vi "Generate ramp lists.vi"(9 "SMU2 settings":T1, 10 "SMU1 settings":T1, 11 "Data in":T2) -> (3 "Data out":T2)   [LabVIEW 2021]
uses:
  controls/MainData.ctl
  <vilib>/Analysis/1siggen.llb/Ramp Pattern by Samples.vi
  <vilib>/Analysis/NI_AALBase.lvlib
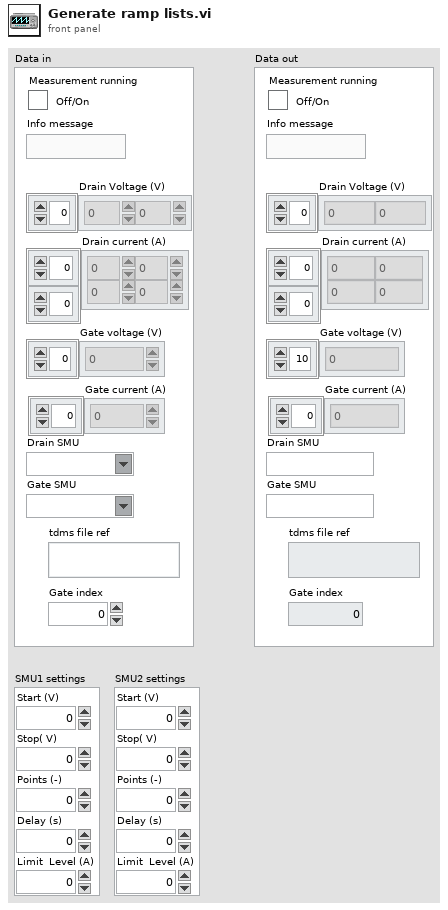
[diagram p1: front panel]
types:
  T1 = cluster{"Start (V) ":dbl, "Stop( V) ":dbl, "Points (-)":u32, "Delay (s)":dbl, "Limit  Level (A)":dbl}
  T2 = typedef "MainData.ctl" = cluster{"Measurement running":bool, "Info message":string, "Drain Voltage (V)":dbl[], "Drain current (A)":dbl[][], "Gate voltage (V)":dbl[], "Gate current (A)":dbl[], "Drain SMU":refnum<visa-resource-name>, "Gate SMU":refnum<visa-resource-name>, "Gate index":i32, "tdms file ref":path}
  T3 = cluster{"Start (V) ":dbl, "Stop( V) ":dbl, "Points (-)":u32, "Delay (s)":dbl, "Limit  Level (A)":dbl}[]
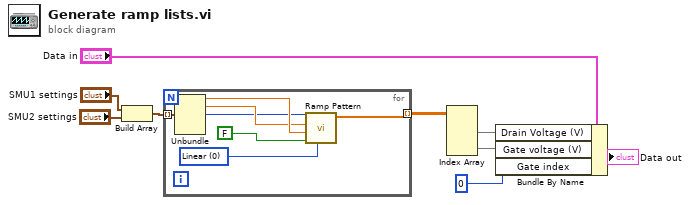
[diagram p0: block diagram]
diagram:
  n1 = Build Array("SMU1 settings", "SMU2 settings") -> (w5:T3)
  n2 = for {
    tunnel: [w16] -> w4 mode=indexing
    tunnel: w5 -> [w10] mode=indexing
    w11 = u16 0 items=["Linear", "Logarithmic"] ("type")
    n3 = Unbundle(w10) -> ("Start (V)"=w14:dbl, "Stop( V)"=w13:dbl, "Points (-)"=w12:u32)  [unwired: 2 out]
    n4 = call-poly <vilib>:"Ramp Pattern.vi"("type"=w11, "exclude end?"=FALSE, "start"=w14, "end"=w13, "samples"=w12) -> ("Ramp Pattern"=w16:dbl[])  [unwired: 5 in, 1 out]
  }
  n5 = Index Array(array=w4) -> (element #1=w3:dbl[], element #2=w2:dbl[])  [unwired: 4 in]
  n6 = Bundle By Name(cluster="Data in", "Drain Voltage (V)"=w3, "Gate voltage (V)"=w2, "Gate index"=0 ("Counter 1")) -> (→"Data out":T2)
